vi "onDestroy.vi"(8 "error in (no error)":errorcluster, 11 "PolyA":refnum<class "ModuleA.lvclass">) -> (0 "error out":errorcluster, 3 "PolyA out":refnum<class "ModuleA.lvclass">)   [LabVIEW 2014, in "ModuleA.lvclass"]
doc: "JKI State Machine Objects (SMO) 1.4.0.57\nJKI - JKI\nCopyright (c) 2018, JKI"
uses:
  ModuleA.lvclass
  ModuleA.lvclass/ModuleA.ctl
  <vilib>/JKI/JKI SMO/SMO/SMO.lvclass
panel:
  # "For instructions on how to use the JKI State Machine Objects, examples and video tutorials, visit:\nhttp://jki.net/state-machine-objects/\n\nJKI State Machine Objects™\nhttp://jki.net/state-machine-objects/\nCopyright (C) 2005-2015, JKI <info@jki.net>\nALL RIGHTS RESERVED"
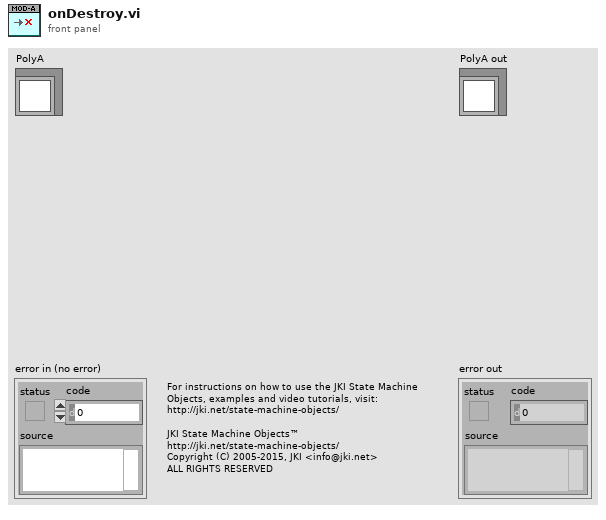
[diagram p1: front panel]
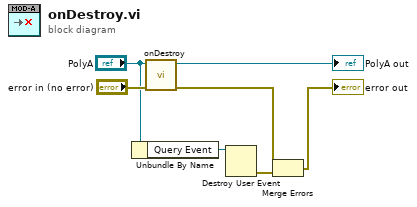
[diagram p0: block diagram]
diagram:
  n1 = Unbundle By Name("PolyA") -> ("Query Event"=w4:refnum<user-event>)
  n2 = call-parent "onDestroy.vi"("error in (no error)"="error in (no error)", "SMO"="PolyA") -> ("error out"=w2:errorcluster, "SMO out"=→"PolyA out":refnum<class "ModuleA.lvclass">)  [unwired: 8 in]
  n3 = Destroy User Event(user event=w4) -> (error out=w3:errorcluster)  [unwired: 1 in]
  n4 = Merge Errors(w2, w3) -> (→"error out":errorcluster)
